vi "Get SMO Database Paths.vi"(5 "getAll Cluster":variant, 7 "Default Paths":string, 8 "error in (no error)":errorcluster, 11 "instrument.PPMS in":refnum<class "instrument.PPMS.lvclass">) -> (0 "error out":errorcluster, 2 "Paths":string, 3 "instrument.PPMS out":refnum<class "instrument.PPMS.lvclass">)   [LabVIEW 2019, in "instrument.PPMS.lvclass"]
uses:
  instrument.PPMS.lvclass
  Typedefs/PPMS.getAll--cluster.ctl
  <userlib>/LevyLab/Instrument Framework/Instrument Types/Cryostat/Instrument.Cryostat.lvclass
  <vilib>/Utility/Data Type/NI_Data Type.lvlib
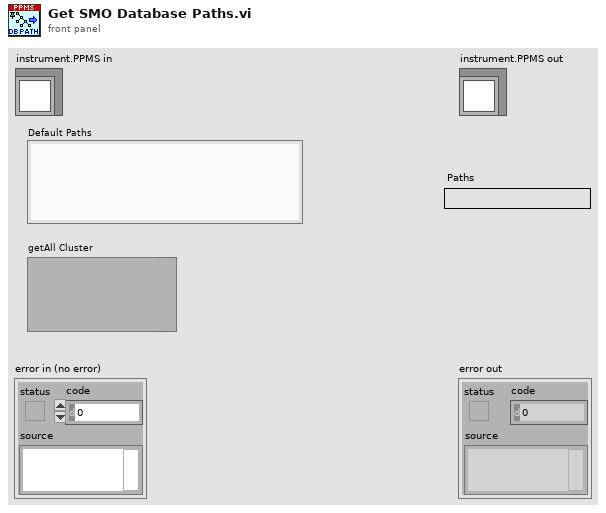
[diagram p1: front panel]
types:
  T1 = typedef "instrument.PPMS.lvclass/PPMS.getAll--cluster.ctl" = cluster{"Chamber Status":string, "Helium Level":dbl, "Temperature":dbl, "Temperature Status":string, "Magnetic Field":dbl, "Magnet Status":string, "Position":dbl}
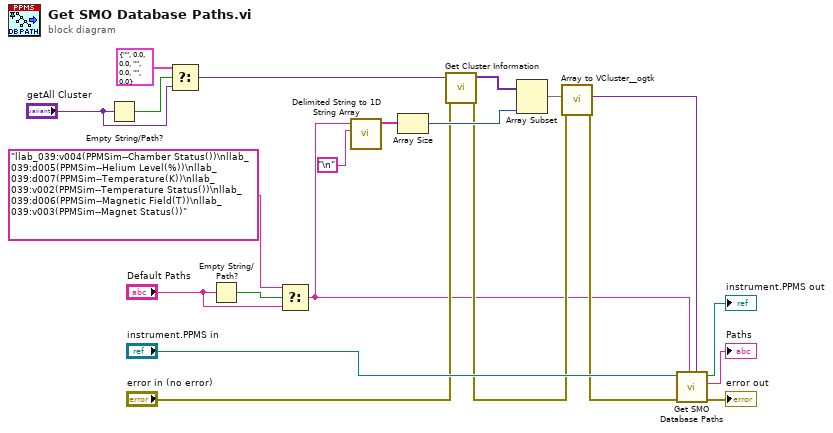
[diagram p0: block diagram]
diagram:
  n1 = Empty String/Path?(string/path="getAll Cluster") -> (empty?=w15:bool)
  n2 = Select(t=T1 {"Chamber Status"="", "Helium Level"=0.0, "Temperature"=0.0, "Temperature Status"="", "Magnetic Field"=0.0, "Magnet Status"="", "Position"=0.0} ("getAll"), s=w15, f="getAll Cluster") -> (s? t:f=w8:variant)
  n3 = Empty String/Path?(string/path="Default Paths") -> (empty?=w17:bool)
  n4 = Select(t="llab_039:v004(PPMSim--Chamber Status())\nllab_039:d005(PPMSim--Helium Level(%))\nllab_039:d007(PPMSim--Temperature(K))\nllab_039:v002(PPMSim--Temperature Status())\nllab_039:d006(PPMSim--Magnetic Field(T))\nllab_039:v003(PPMSim--Magnet Status())" ("Paths"), s=w17, f="Default Paths") -> (s? t:f=w1:string)
  n5 = call <vilib>:"Delimited String to 1D String Array.vi"("delimiter"="\n", "delimited string"=w1) -> ("string array"=w11:string[])  [unwired: 9 in]
  n6 = Array Size(array=w11) -> (size(s)=w6:i32)
  n7 = call <vilib>:"Get Cluster Information.vi"("error in (no error)"="error in (no error)", "variant"=w8) -> ("error out"=w4:errorcluster, "cluster elements"=w12:variant[])  [unwired: 8 in]
  n8 = Array Subset(array=w12, length=w6) -> (w9:variant[])  [unwired: 1 in]
  n9 = call <userlib>:"Array to VCluster__ogtk.vi"("error in (no error)"=w4, "Array"=w9) -> ("error out"=w3:errorcluster, "VCluster"=w7:variant)  [unwired: 8 in]
  n10 = call-parent "Get SMO Database Paths.vi"("getAll Cluster"=w7, "Default Paths"=w1, "error in (no error)"=w3, "Instrument in"="instrument.PPMS in") -> ("error out"=→"error out":errorcluster, "Paths"=→"Paths":string, "Instrument out"=→"instrument.PPMS out":refnum<class "instrument.PPMS.lvclass">)  [unwired: 5 in]
